vi "Set Show Sent Messages.vi"(8 "error in (no error)":errorcluster, 10 "Show Sent Messages?":bool, 11 "Debug Log View In":refnum<class "Debug Log View.lvclass">) -> (0 "error out":errorcluster, 3 "Debug Log View Out":refnum<class "Debug Log View.lvclass">)   [LabVIEW 2020, in "Debug Log View.lvclass"]
uses:
  Debug Log View.lvclass
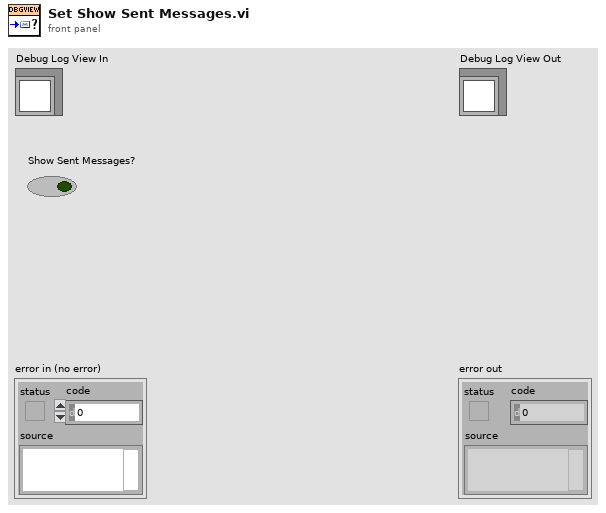
[diagram p1: front panel]
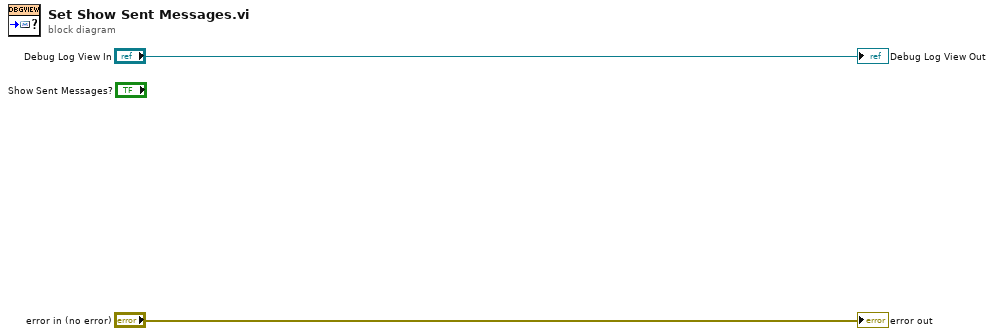
[diagram p0: block diagram]
diagram:
  "error out" <- "error in (no error)"
  "Debug Log View Out" <- "Debug Log View In"
